vi "save.vi"(4 "log?":bool, 8 "data":dbl[](array[numeric]), 11 "Qube":refnum<class "Qube.lvclass">) -> (3 "Qube":refnum<class "Qube.lvclass">)   [LabVIEW 2017, in "Qube.lvclass"]
uses:
  Qube.lvclass
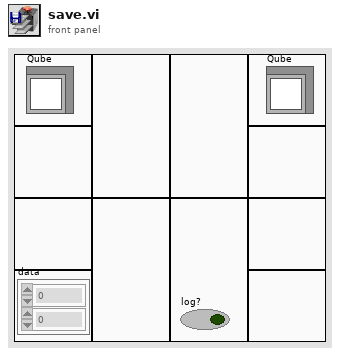
[diagram p1: front panel]
types:
  T1 = enum16{"big-endian, network order", "native, host order", "little-endian"}
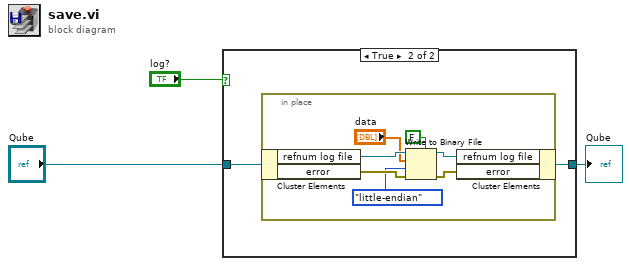
[diagram p0: block diagram]
diagram:
  n1 = case shown="True" "log?" {
    tunnel: "Qube" -> [w4 w6]
    tunnel: [w4 w5] -> w1
    frame False {
    }
    frame True {
      n2 = in-place {
        n3 = in-place-cluster #1(w6) -> ("refnum log file"=w13:refnum<file>, "error"=w11:errorcluster)
        n4 = Write to Binary File(file (use dialog)=w13, data="data", error in=w11, 5:FALSE ("prepend array or string size? (T)"), 9:T1."little-endian" ("byte order (0:big-endian, network order)")) -> (refnum out=w12:refnum<file>, error out=w10:errorcluster)  [unwired: 1 in, 1 out]
        n5 = in-place-cluster #1("refnum log file"=w12, "error"=w10) -> (w5:refnum<class "Qube.lvclass">)
      }
    }
  }
  "Qube" <- w1
